vi "Open File.vi"(8 "error in":errorcluster, 11 "TDMS in":refnum<class "TDMS.lvclass">) -> (0 "error out":errorcluster, 3 "TDMS out":refnum<class "TDMS.lvclass">)   [LabVIEW 2020, in "Manejador archivo.lvlib" / "TDMS.lvclass"]
uses:
  TDMS.lvclass
  C:/GitClones/DQMH-LabVIEW-GYM/10 Mayo/04 DQMH USER/Libraries/Manejador archivo/Class Definitions/File/File.lvclass
  TDMS.lvclass/TDMS.ctl
  File/File.lvclass/File.ctl
  File/Read File Path.vi
  Write tdms file ref.vi
  Read tdms file ref.vi
  File/File.lvclass
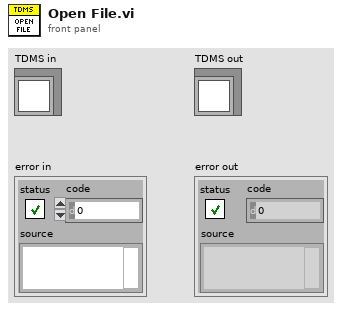
[diagram p1: front panel]
types:
  T1 = enum16{"open", "open or create", "create or replace", "create", "open (read-only)"}
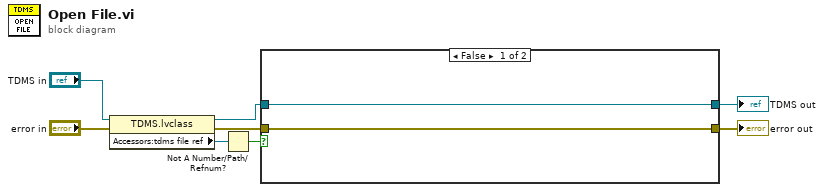
[diagram p0: block diagram]
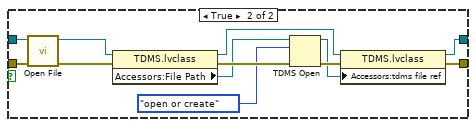
[diagram p2: hidden frame]
diagram:
  n1 = property class="TDMS.lvclass"(reference="TDMS in", error in="error in") -> (reference out=w3:refnum<class "TDMS.lvclass">, error out=w6:errorcluster, "Accessors:tdms file ref"=w2:refnum<k34>)
  n2 = Not A Number/Path/Refnum?(number/path/refnum=w2) -> (NaN/Path/Refnum?=w1:bool)
  n3 = case shown="False" w1 {
    tunnel: w6 -> [w10 w22]
    tunnel: [w10 w19] -> w7
    tunnel: w3 -> [w9 w12]
    tunnel: [w9 w14] -> w5
    frame False {
    }
    frame True {
      n4 = call-parent "Open File.vi"("error in"=w22, "File in"=w12) -> ("error out"=w18:errorcluster, "File out"=w11:refnum<class "TDMS.lvclass">)  [unwired: 8 in]
      n5 = property class="TDMS.lvclass"(reference=w11, error in=w18) -> (reference out=w15:refnum<class "TDMS.lvclass">, error out=w21:errorcluster, "Accessors:File Path"=w17:path)
      n6 = TDMS Open(8:w21, 10:T1."open or create" ("operation (0:open)"), 11:w17) -> (0:w20:errorcluster, 3:w13:refnum<k34>)  [unwired: 4 in]
      n7 = property class="TDMS.lvclass"(reference=w15, error in=w20, "Accessors:tdms file ref"=w13) -> (reference out=w14:refnum<class "TDMS.lvclass">, error out=w19:errorcluster)
    }
  }
  "error out" <- w7
  "TDMS out" <- w5
